vi "sub vi - cycle&temp fail v7.vi"(0 "Amps Lo?":bool, 2 "Input Cluster":T1, 3 "SELECT":T2(ring), 4 "Amps Hi?":bool, 5 "Result In":bool, 8 "Panel":u64) -> (15 "(FAIL) out":cluster{"FAIL LO":dbl, "FAIL HI":dbl}, 16 "(DISP) out":T3, 17 "T-RISE":cluster{"T-RISE (L)":dbl, "T-RISE (N)":dbl}, 18 "Result Out":bool, 19 "file error":errorcluster)   [LabVIEW 2017]
uses:
  program files/Global display 3.vi
  program files/Global 1.vi
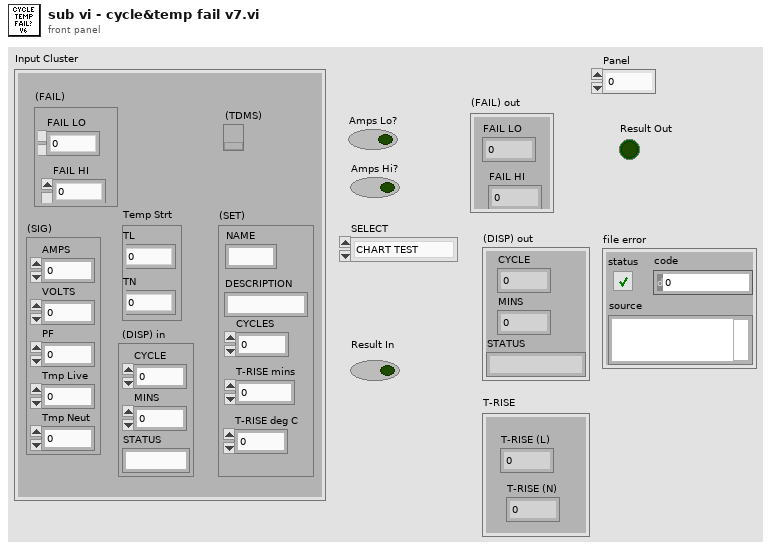
[diagram p1: front panel]
types:
  T1 = cluster{"(FAIL)":cluster{"FAIL LO":dbl, "FAIL HI":dbl}, "(SIG)":cluster{"AMPS":dbl, "VOLTS":dbl, "PF":dbl, "Tmp Live":dbl, "Tmp Neut":dbl}, "Temp Strt":cluster{"TL":dbl, "TN":dbl}, " (DISP) in":cluster{"CYCLE":dbl, "MINS":dbl, "STATUS":string}, "(SET)":cluster{"NAME":string, "DESCRIPTION":string, "CYCLES":dbl, "T-RISE mins":dbl, "T-RISE deg C":dbl}, "(TDMS)":refnum<k34>}
  T2 = enum32{"CHART TEST", "CYCLE TEST", "T-RISE TEST"}
  T3 = cluster{"CYCLE":dbl, "MINS":dbl, "STATUS":string}
  T4 = cluster{"AMPS":dbl, "VOLTS":dbl, "PF":dbl, "Tmp Live":dbl, "Tmp Neut":dbl}
  T5 = cluster{"NAME":string, "DESCRIPTION":string, "CYCLES":dbl, "T-RISE mins":dbl, "T-RISE deg C":dbl}
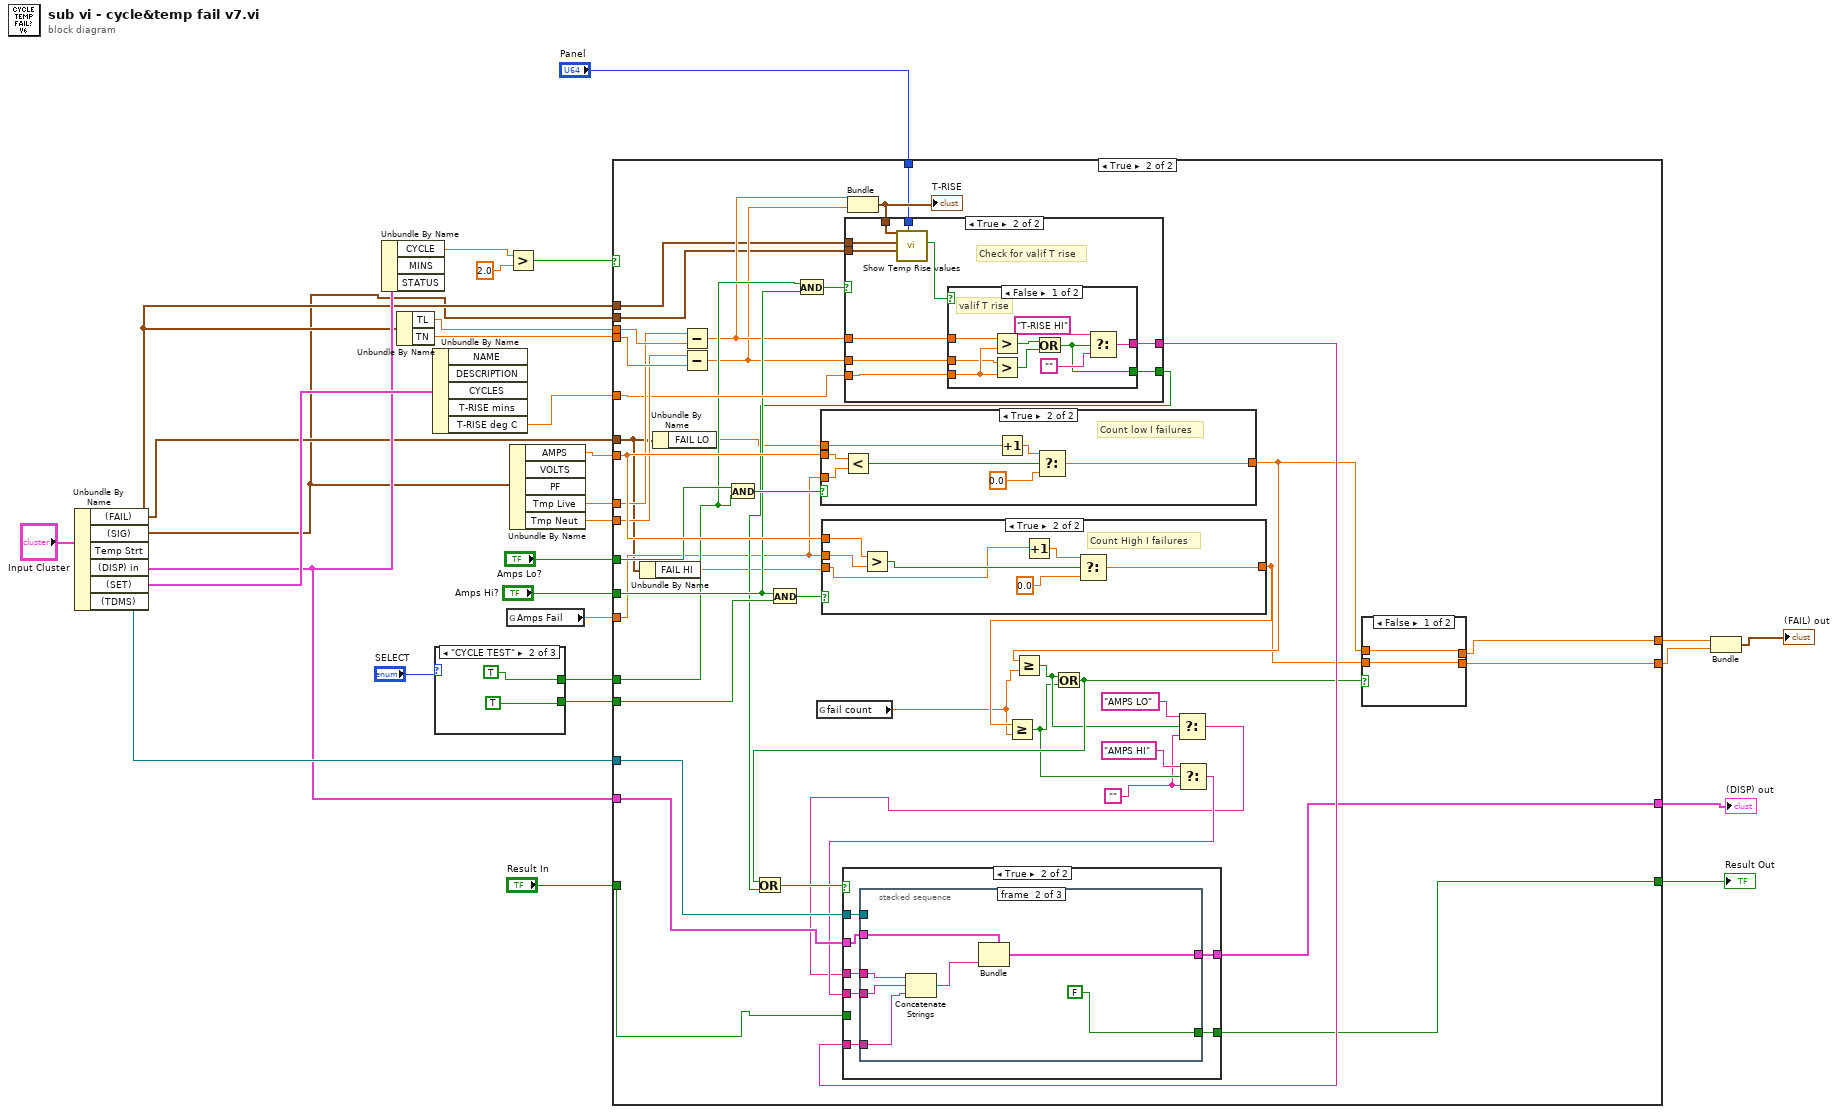
[diagram p0: block diagram]
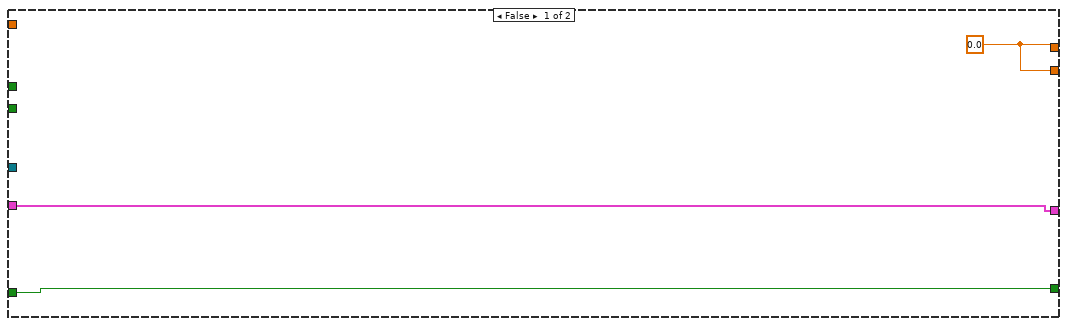
[diagram p2: hidden frame]
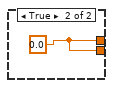
[diagram p3: hidden frame]
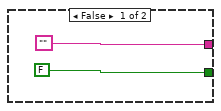
[diagram p4: hidden frame]
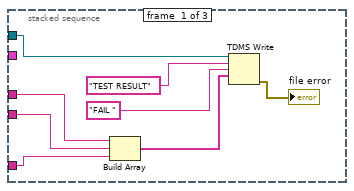
[diagram p7: hidden frame]
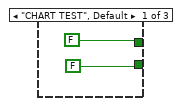
[diagram p11: hidden frame]
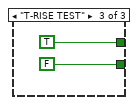
[diagram p12: hidden frame]
diagram:
  n1 = Unbundle By Name("Input Cluster") -> ("(FAIL)"=w4:cluster{"FAIL LO":dbl, "FAIL HI":dbl}, "(SIG)"=w2:T4, "Temp Strt"=w3:cluster{"TL":dbl, "TN":dbl}, "(DISP) in"=w9:T3, "(SET)"=w17:T5, "(TDMS)"=w16:refnum<k34>)
  n2 = Unbundle By Name(w9) -> ("CYCLE"=w8:dbl)  [unwired: 2 out]
  n3 = Unbundle By Name(w3) -> ("TL"=w6:dbl, "TN"=w5:dbl)
  n4 = Unbundle By Name(w17) -> ("T-RISE deg C"=w25:dbl)  [unwired: 4 out]
  n5 = case shown="\"CYCLE TEST\"" "SELECT" {
    tunnel: [FALSE TRUE TRUE] -> w21
    tunnel: [FALSE TRUE FALSE] -> w24
    frame "CHART TEST", Default {
    }
    frame "CYCLE TEST" {
    }
    frame "T-RISE TEST" {
    }
  }
  n6 = global read "Global display 3.vi" "Amps Fail"() -> (w7:dbl)
  n7 = Greater?(x=w8, y=2.0) -> (0:w19:bool)
  n8 = Unbundle By Name(w2) -> ("AMPS"=w28:dbl, "Tmp Live"=w27:dbl, "Tmp Neut"=w26:dbl)  [unwired: 2 out]
  n9 = case shown="True" w19 {
    tunnel: w28 -> [_ w82]
    tunnel: w16 -> [_ w81]
    tunnel: w9 -> [w37 w80]
    tunnel: w6 -> [_ w79]
    tunnel: w5 -> [_ w78]
    tunnel: w27 -> [_ w77]
    tunnel: w26 -> [_ w76]
    tunnel: w25 -> [_ w75]
    tunnel: w24 -> [_ w72]
    tunnel: "Amps Lo?" -> [_ w70]
    tunnel: "Amps Hi?" -> [_ w68]
    tunnel: w21 -> [_ w67]
    tunnel: [w38 w64] -> w14
    tunnel: [w38 w63] -> w13
    tunnel: [w37 w62] -> w12
    tunnel: [w36 w61] -> w11
    tunnel: "Result In" -> [w36 w60]
    tunnel: w7 -> [_ w46]
    tunnel: w4 -> [_ w44]
    tunnel: w3 -> [_ w42]
    tunnel: w2 -> [_ w41]
    tunnel: "Panel" -> [_ w39]
    frame False {
      w38 = 0.0
    }
    frame True {
      w52 = ""
      n10 = Unbundle By Name(w44) -> ("FAIL HI"=w43:dbl)
      n11 = Unbundle By Name(w44) -> ("FAIL LO"=w45:dbl)
      n12 = Subtract(x=w77, y=w79) -> (x-y=w49:dbl)
      n13 = Subtract(x=w76, y=w78) -> (x-y=w48:dbl)
      n14 = And(x=w70, y=w67) -> (x .and. y?=w71:bool)
      n15 = And(x=w68, y=w72) -> (x .and. y?=w73:bool)
      n16 = And(x=w67, y=w68) -> (x .and. y?=w69:bool)
      n17 = global read "Global 1.vi" "fail count"() -> (w47:dbl)
      n18 = case shown="True" w71 {
        tunnel: w82 -> [_ w146]
        tunnel: w46 -> [_ w145]
        tunnel: w45 -> [w139 w141]
        tunnel: [w139 w140] -> w66
        frame False {
        }
        frame True {
          # "Count low I failures"
          n19 = Less?(x=w146, y=w145) -> (x < y?=w144:bool)
          n20 = Increment(x=w141) -> (x+1=w143:dbl)
          n21 = Select(t=w143, s=w144, f=0.0) -> (s? t:f=w140:dbl)
        }
      }
      n22 = case shown="True" w73 {
        tunnel: w82 -> [_ w138]
        tunnel: w46 -> [_ w137]
        tunnel: [w131 w133] -> w65
        tunnel: w43 -> [w131 w132]
        frame False {
        }
        frame True {
          # "Count High I failures"
          n23 = Greater?(x=w138, y=w137) -> (0:w136:bool)
          n24 = Increment(x=w132) -> (x+1=w135:dbl)
          n25 = Select(t=w135, s=w136, f=0.0) -> (s? t:f=w133:dbl)
        }
      }
      n26 = Bundle(w49, w48) -> (w40:cluster{dbl, dbl})  [unwired: 1 in]
      "T-RISE" <- w40
      n27 = case shown="True" w69 {
        tunnel: w75 -> [_ w97]
        tunnel: w49 -> [_ w94]
        tunnel: w48 -> [_ w93]
        tunnel: ["" w96] -> w74
        tunnel: [FALSE w95] -> w58
        tunnel: w42 -> [_ w92]
        tunnel: w41 -> [_ w91]
        tunnel: w40 -> [_ w90]
        tunnel: w39 -> [_ w88]
        frame False {
        }
        frame True {
          # "Check for valif T rise"
          n28 = call "Show Temp Rise values.vi"("Panel"=w88, "(SIG) in"=w91, "Temp Strt in"=w92, "T Rise"=w90) -> ("Invalid T Rise"=w89:bool)  [unwired: 7 in]
          n29 = case shown="False" w89 {
            tunnel: w97 -> [w106 _]
            tunnel: [w101 _] -> w96
            tunnel: [w100 _] -> w95
            tunnel: w94 -> [w99 _]
            tunnel: w93 -> [w98 _]
            frame False {
              # "valif T rise"
              n30 = Greater?(x=w99, y=w106) -> (0:w104:bool)
              n31 = Greater?(x=w98, y=w106) -> (0:w105:bool)
              n32 = Or(x=w104, y=w105) -> (x .or. y?=w100:bool)
              n33 = Select(t="T-RISE HI", s=w100, f="") -> (s? t:f=w101:string)
            }
            frame True {
            }
          }
        }
      }
      n34 = Greater Or Equal?(x=w65, y=w47) -> (x >= y?=w55:bool)
      n35 = Greater Or Equal?(x=w66, y=w47) -> (x >= y?=w56:bool)
      n36 = Or(x=w56, y=w55) -> (x .or. y?=w59:bool)
      n37 = Or(x=w59, y=w58) -> (x .or. y?=w57:bool)
      n38 = Select(t="AMPS LO", s=w56, f=w52) -> (s? t:f=w50:string)
      n39 = Select(t="AMPS HI", s=w55, f=w52) -> (s? t:f=w51:string)
      n40 = case shown="True" w57 {
        tunnel: w50 -> [_ w115]
        tunnel: w51 -> [_ w114]
        tunnel: w80 -> [w108 w113]
        tunnel: w81 -> [_ w112]
        tunnel: w74 -> [_ w111]
        tunnel: [w108 w110] -> w62
        tunnel: [w107 w109] -> w61
        tunnel: w60 -> [w107 _]
        frame False {
        }
        frame True {
          n41 = stacked-sequence {
            tunnel: w115 -> [w116 w130 _]
            tunnel: w114 -> [w117 w129 _]
            tunnel: w113 -> [_ w127 _]
            tunnel: w112 -> [w119 _ _]
            tunnel: w111 -> [w118 w126 _]
            tunnel: [_ w125 _] -> w110
            tunnel: [_ FALSE _] -> w109
            frame #0 {
              n42 = Build Array(w116, w117, w118) -> (w122:string[])
              n43 = TDMS Write(0:w119, 5:"TEST RESULT", 7:"FAIL ", 9:w122) -> (15:→"file error":errorcluster)  [unwired: 2 in, 3 out]
            }
            frame #1 {
              n44 = Concatenate Strings(w130, w129, w126) -> (w128:string)
              n45 = Bundle(cluster=w127, "STATUS"=w128) -> (w125:T3)  [unwired: 2 in]
            }
            frame #2 {
            }
          }
        }
      }
      n46 = case shown="False" w59 {
        tunnel: w66 -> [w84 _]
        tunnel: w65 -> [w83 _]
        tunnel: [w84 w85] -> w64
        tunnel: [w83 w85] -> w63
        frame False {
        }
        frame True {
          w85 = 0.0
        }
      }
    }
  }
  "(DISP) out" <- w12
  "Result Out" <- w11
  n47 = Bundle("FAIL LO"=w14, "FAIL HI"=w13) -> (→"(FAIL) out":cluster{"FAIL LO":dbl, "FAIL HI":dbl})  [unwired: 1 in]
